vi "MyAnd.vi"(9 "Y":bool, 10 "X":bool) -> (2 "X and Y":bool)   [LabVIEW 2020]
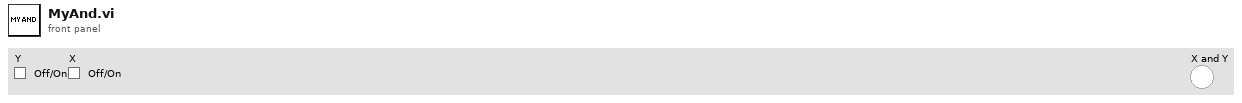
[diagram p1: front panel]
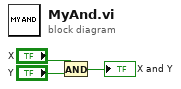
[diagram p0: block diagram]
diagram:
  n1 = And(x="X", y="Y") -> (x .and. y?=→"X and Y":bool)
